vi "Host Main.vi"() -> ()   [LabVIEW 2017]
doc: "This application launches and executes the Tag Bus Data framework configuration for the specified target alias. This is a simple example of the framework API functions, but may also be a suitable starting point for a Host UI or Thick Client that is running a local version of the framework."
uses:
  <vilib>/NI/Module Execution Interface/Engine Runtime/Execution States.ctl
  <vilib>/NI/Module Execution Interface/Engine Runtime/Fault.ctl
  <vilib>/NI/Tag Bus Module Framework/runtime/error classification.ctl
  <vilib>/userdefined/High Color/nirio_resource_hc.ctl
  <vilib>/NI/DCAF/addons/InstructionFrameworkSupport/FPGA_FGV_action.ctl
  <vilib>/NI/Current Value Table/DataTypes/Double_Read.vi
  <vilib>/NI/Current Value Table/DataTypes/Boolean_Read.vi
  <vilib>/NI/Current Value Table/Type to Enum.vi
  <vilib>/NI/Current Value Table/DataTypes/Double_Type To Enum.vi
  <vilib>/NI/Current Value Table/DataTypes/Boolean_Type To Enum.vi
  <vilib>/FPGAPlugInAG/sbRIO-9607/niLvFpga_Open_sbRIO-9607.vi
  <vilib>/rvi/interface/common/dynamic/niFpgaDynamicAddResources.vi
  <vilib>/NI/Current Value Table/FGVs/CVT Globals.vi
  <vilib>/NI/Current Value Table/FGVs/Tag Memory.vi
  <vilib>/NI/Current Value Table/Memory Block.vi
  <vilib>/NI/Current Value Table/DataTypes/Boolean_Memory Block.vi
  <vilib>/NI/Current Value Table/DataTypes/Double_Memory Block.vi
  <vilib>/rvi/interface/nirviOpenFPGA/nirviOpenFPGA.xnode
  FPGA Bitfiles/ThreePhaseDevEng_FPGATarget_Firmware_Px3FQXq-HBM.lvbitx
  <vilib>/NI/Module Execution Interface/Engine Runtime/Engine Runtime Interface.lvclass
  <vilib>/NI/DCAF/Tag Editor Core/Framework Configuration Classes/target runtime/PL_Target Runtime.lvclass
  <vilib>/NI/Tag Bus Module Framework/FPGA manager/FPGA manager.lvlib
  <vilib>/NI/Tag Bus Module Framework/FPGA manager/methods.ctl
  <vilib>/NI/Tag Bus Module Framework/runtime/TBM module execution interface.lvclass
  <vilib>/NI/Current Value Table/Current Value Table.lvlib
panel:
  out "detectedFreq":dbl
  out "Locked":bool
  out "engine status":T4(array[cluster])
  in  "stop":bool
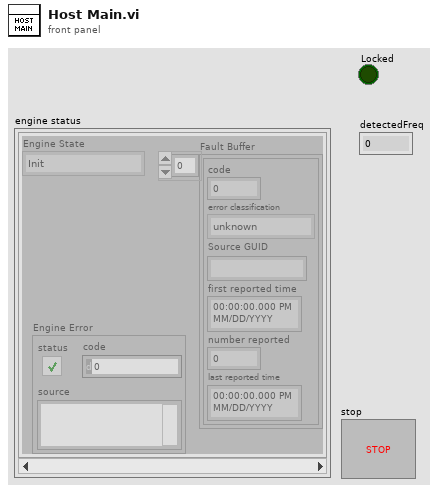
[diagram p1: front panel]
types:
  T1 = typedef "Engine Runtime Interface.lvclass/Execution States.ctl" = enum16{"Init", "Pre-Operational", "Safe-Operational", "Operational", "Stopped"}
  T2 = typedef "Engine Runtime Interface.lvclass/Fault.ctl" = cluster{"code":i32, "error classification":T3, "Source GUID":string, "first reported time":timestamp, "number reported":u32, "last reported time":timestamp}
  T3 = typedef "TBM module execution interface.lvclass/error classification.ctl" = enum16{"unknown", "none", "trivial", "recoverable", "critical"}
  T4 = cluster{"Engine State":T1, "Fault Buffer":T2[], "Engine Error":errorcluster}[]
  T5 = typedef "FPGA_FGV_action.ctl" = enum16{"get FPGA", "set FPGA", "Close"}
  T6 = typedef "nirio_resource_hc.ctl" = tag
  T7 = cluster{"Engine State":T1, "Fault Buffer":T2[], "Engine Error":errorcluster}
  T8 = typedef "FPGA manager.lvlib/methods.ctl" = enum16{"initialize bitfile", "cache bitfile", "locate bitfile", "close bitfile", "clear manager"}
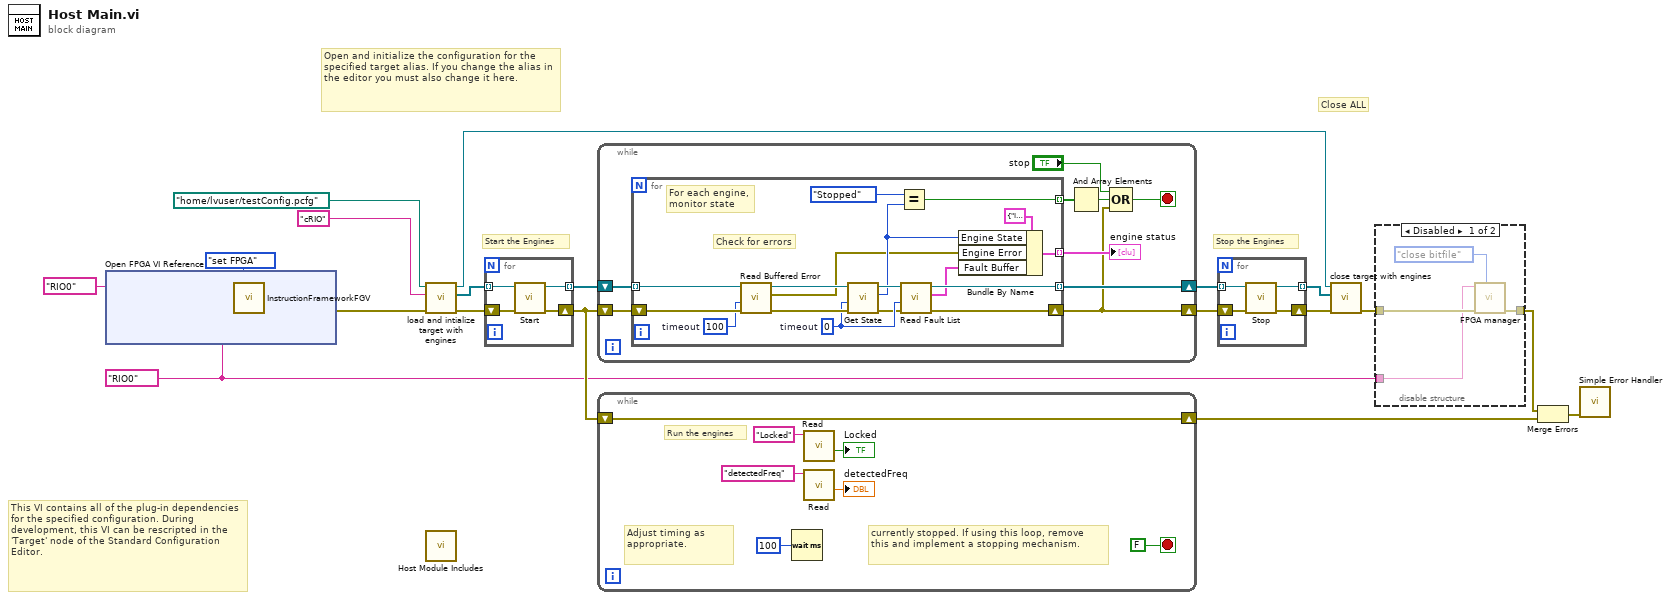
[diagram p0: block diagram]
diagram:
  w5 = T6 "RIO0" ("RIO resource")
  # "Start the Engines"
  # "Open and initialize the configuration for the specified target alias. If you change the alias in the editor you must also change it here."
  # "Close ALL"
  # "Stop the Engines"
  # "This VI contains all of the plug-in dependencies for the specified configuration. During development, this VI can be rescripted in the 'Target' node of the Standard Configuration Editor."
  # "Run the engines"
  n1 = xnode "Open FPGA VI Reference"("resource name"=tag "RIO0") -> ("FPGA VI Reference Out"=w6:refnum<k20>, "error out"=w4:errorcluster)  [unwired: 1 in]
  n2 = call <vilib>:"InstructionFrameworkFGV.vi"("RIO resource"=w5, "Action"=FPGA_FGV_action."set FPGA", "bitfile to cache"=w6, "error in"=w4) -> ("error out"=w3:errorcluster)  [unwired: 9 in, 2 out]
  n3 = call <vilib>:"load and intialize target with engines.vi"("error in"=w3, "target alias"="cRIO", "file path"=path "/home/lvuser/testConfig.pcfg" ("configuration file path")) -> ("error out"=w18:errorcluster, "engine runtime interfaces"=w17:refnum<class "Engine Runtime Interface.lvclass">[], "target runtime"=w14:refnum<class "PL_Target Runtime.lvclass">)  [unwired: 6 in]
  n4 = call "Host Module Includes.vi"() -> ()  [unwired: 12 in]
  n5 = for {
    tunnel: [w25] -> w21 mode=indexing
    tunnel: w17 -> [w22] mode=indexing
    shift-right: [w24] -> w12
    shift-left: w18 -> [w23]
    n6 = call-dynamic "Start.vi"("error in"=w23, "Engine Runtime Interface in"=w22) -> ("error out"=w24:errorcluster, "Engine Runtime Interface out"=w25:refnum<class "Engine Runtime Interface.lvclass">)  [unwired: 8 in]
  }
  n7 = while {
    shift-right: [w32] -> w20
    shift-left: w21 -> [w34]
    shift-right: [w26] -> w19
    shift-left: w12 -> [w33]
    stop <- w30 stop-if-true
    n8 = for {
      tunnel: w34 -> [w51] mode=indexing
      tunnel: [w43] -> w32 mode=indexing
      tunnel: [w46] -> w28 mode=indexing
      shift-right: [w42] -> w26
      shift-left: w33 -> [w50]
      tunnel: [w38] -> w29 mode=indexing
      w41 = 0  # timeout
      w45 = 100  # timeout
      # "For each engine, \nmonitor state"
      # "Check for errors"
      n9 = call-dynamic "Read Buffered Error.vi"("error in"=w50, "timeout in ms (0)"=w45, "Engine Runtime Interface in"=w51) -> ("error out"=w48:errorcluster, "Engine Error"=w36:errorcluster, "Engine Runtime Interface out"=w49:refnum<class "Engine Runtime Interface.lvclass">)  [unwired: 6 in]
      n10 = call-dynamic "Get State.vi"("error in"=w48, "timeout (-1)"=w41, "Engine Runtime Interface in"=w49) -> ("error out"=w35:errorcluster, "Engine State"=w40:T1, "Engine Runtime Interface out"=w44:refnum<class "Engine Runtime Interface.lvclass">)  [unwired: 6 in]
      n11 = Equal?(x=Execution_States."Stopped" ("Engine State"), y=w40) -> (x = y?=w46:bool)
      n12 = call-dynamic "Read Fault List.vi"("error in"=w35, "timeout (-1)"=w41, "Engine Runtime Interface in"=w44) -> ("error out"=w42:errorcluster, "faults"=w39:T2[], "Engine Runtime Interface out"=w43:refnum<class "Engine Runtime Interface.lvclass">)  [unwired: 6 in]
      n13 = Bundle By Name(cluster=T7 {"Engine State"=enum."Init", "Fault Buffer"=[], "Engine Error"={"status"=FALSE, "code"=0, "source"=""}}, "Engine State"=w40, "Engine Error"=w36, "Fault Buffer"=w39) -> (w38:T7)
    }
    "engine status" <- w29
    n14 = And Array Elements(Boolean array=w28) -> (logical AND=w27:bool)
    n15 = Compound Arithmetic op=OR("stop", w27, w26) -> (w30:bool)
  }
  n16 = while {
    shift-right: [w56] -> w11
    shift-left: w12 -> [w56]
    stop <- FALSE stop-if-true
    # "currently stopped. If using this loop, remove \nthis and implement a stopping mechanism."
    # "Adjust timing as appropriate."
    n17 = Wait (ms)(milliseconds to wait=u32 100) -> ()  [unwired: 1 out]
    n18 = call-poly <vilib>:"Read.vi"("Tag Name"="Locked") -> ("Value"=→"Locked":bool)  [unwired: 9 in, 1 out]
    n19 = call-poly <vilib>:"Read.vi"("Tag Name"="detectedFreq") -> ("Value"=→"detectedFreq":dbl)  [unwired: 9 in, 1 out]
  }
  n20 = for {
    tunnel: w20 -> [w62] mode=indexing
    shift-right: [w59] -> w13
    shift-left: w19 -> [w61]
    tunnel: [w60] -> w15 mode=indexing
    n21 = call-dynamic "Stop.vi"("error in"=w61, "Engine Runtime Interface in"=w62) -> ("error out"=w59:errorcluster, "Engine Runtime Interface out"=w60:refnum<class "Engine Runtime Interface.lvclass">)  [unwired: 8 in]
  }
  n22 = call <vilib>:"close target with engines.vi"("error in"=w13, "Engine Runtime Interfaces"=w15, "Target Runtime"=w14) -> ("error out"=w10:errorcluster)  [unwired: 8 in]
  n23 = disable-structure shown="Disabled" {
    disable-tunnel: [w65 w67] -> w9
    disable-tunnel: w10 -> [w66 w67]
    disable-tunnel: w5 -> [w63 _]
    frame Disabled {
      n24 = call <vilib>:"FPGA manager.vi"("action"=methods."close bitfile", "error in"=w66, "RIO resource"=w63) -> ("error out"=w65:errorcluster)  [unwired: 6 in, 2 out]
    }
    frame Enabled {
    }
  }
  n25 = Merge Errors(w9, w11) -> (w8:errorcluster)
  n26 = call <vilib>:"Simple Error Handler.vi"("error in (no error)"=w8) -> ()  [unwired: 4 in, 5 out]
